vi "enable.Position.vi"(7 "bus":T1, 8 "error in":errorcluster) -> (0 "error out":errorcluster)   [LabVIEW 2020]
uses:
  bus.ctl
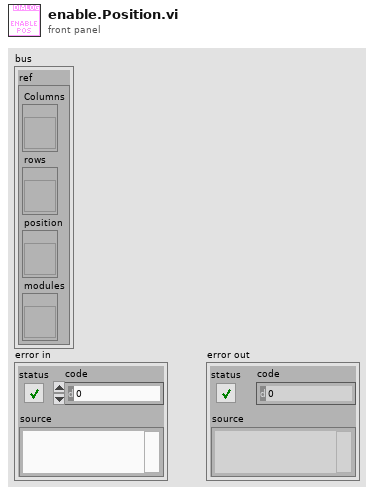
[diagram p1: front panel]
types:
  T1 = typedef "bus.ctl" = cluster{"ref":cluster{"Columns":refnum<vi>, "rows":refnum<vi>, "position":refnum<vi>, "modules":refnum<vi>}}
  T2 = enum8{"Enabled", "Disabled", "Disabled and Grayed Out"}
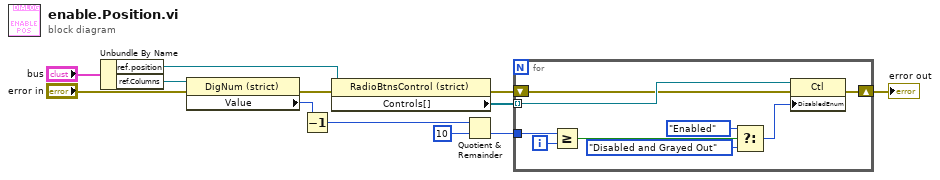
[diagram p0: block diagram]
diagram:
  n1 = Unbundle By Name("bus") -> ("ref.position"=w6:refnum<vi>, "ref.Columns"=w2:refnum<vi>)
  n2 = property on="Property Node" class="DigNum (strict)"(reference=w2) -> ("Value"=w1:u8)  [unwired: 1 in, 2 out]
  n3 = Decrement(x=w1) -> (x-1=w11:u8)
  n4 = property on="Property Node" class="RadioBtnsControl (strict)"(reference=w6, error in="error in") -> (error out=w3:errorcluster, "Controls[]"=w8:refnum<vi>[])  [unwired: 1 out]
  n5 = Quotient & Remainder(x=w11, y=u8 10) -> (floor(x/y)=w10:u8)  [unwired: 1 out]
  n6 = for {
    tunnel: w8 -> [w20] mode=indexing
    tunnel: w10 -> [w19]
    shift-right: [w13] -> w4
    shift-left: w3 -> [w12]
    i -> [w14]
    n7 = Greater Or Equal?(x=w19, y=w14) -> (x >= y?=w18:bool)
    n8 = Select(t=T2."Enabled" ("Disabled"), s=w18, f=T2."Disabled and Grayed Out") -> (s? t:f=w15:T2)
    n9 = property class="Ctl"(reference=w20, error in=w12, "DisabledEnum"=w15) -> (error out=w13:errorcluster)  [unwired: 1 out]
  }
  "error out" <- w4
